vi "comicvine.to.local_issue.vi"(8 "error in (no error)":errorcluster, 11 "cv_issue":T5) -> (0 "error out":errorcluster, 3 "local_issue":T1)   [LabVIEW 2024]
uses:
  definitions/comicvine_issue.ctl
  definitions/comicvine_issue.results.ctl
  definitions/comicvine_issue.associated_image.ctl
  definitions/comicvine_issue.generic_credit.ctl
  definitions/comicvine_issue.person_credit.ctl
  definitions/local_issue.ctl
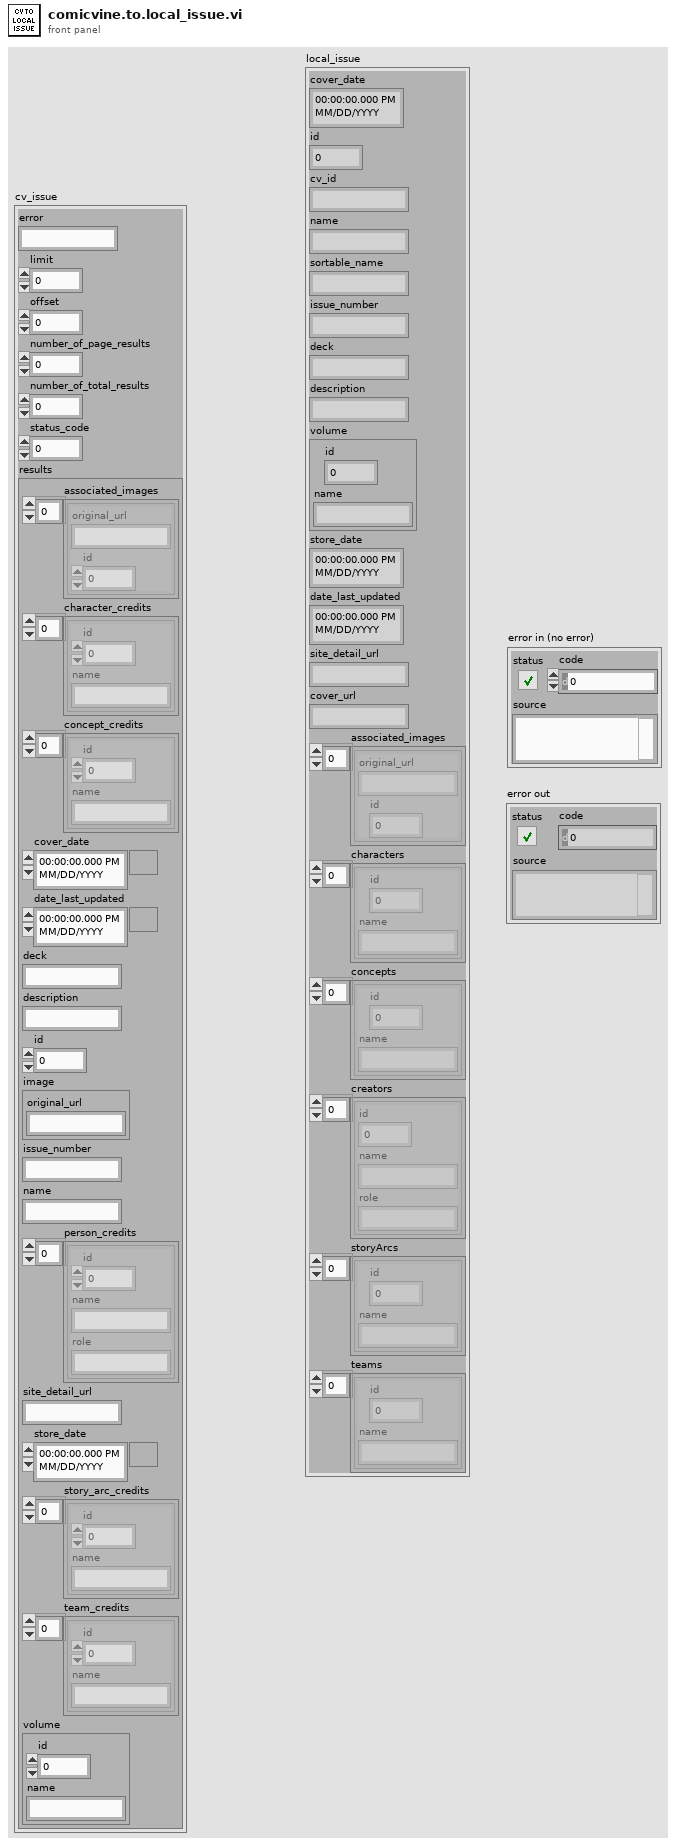
[diagram p1: front panel]
types:
  T1 = typedef "local_issue.ctl" = cluster{"cover_date":timestamp, "id":i32, "cv_id":string, "name":string, "sortable_name":string, "issue_number":string, "deck":string, "description":string, "volume":T2, "store_date":timestamp, "date_last_updated":timestamp, "site_detail_url":string, "cover_url":string, "associated_images":T3[], "characters":T2[], "concepts":T2[], "creators":T4[], "storyArcs":T2[], "teams":T2[]}
  T2 = typedef "comicvine_issue.generic_credit.ctl" = cluster{"id":i32, "name":string}
  T3 = typedef "comicvine_issue.associated_image.ctl" = cluster{"original_url":string, "id":i32}
  T4 = typedef "comicvine_issue.person_credit.ctl" = cluster{"id":i32, "name":string, "role":string}
  T5 = typedef "comicvine_issue.ctl" = cluster{"error":string, "limit":i32, "offset":i32, "number_of_page_results":i32, "number_of_total_results":i32, "status_code":i32, "results":T6}
  T6 = typedef "comicvine_issue.results.ctl" = cluster{"associated_images":T3[], "character_credits":T2[], "concept_credits":T2[], "cover_date":timestamp, "date_last_updated":timestamp, "deck":string, "description":string, "id":i32, "image":cluster{"original_url":string}, "issue_number":string, "name":string, "person_credits":T4[], "site_detail_url":string, "store_date":timestamp, "story_arc_credits":T2[], "team_credits":T2[], "volume":T2}
  T7 = typedef "LVDateTimeRec.ctl" = cluster{"fractional second":dbl, "second":i32, "minute":i32, "hour":i32, "day of month":i32, "month":i32, "year":i32, "day of week":i32, "day of year":i32, "DST":i32}
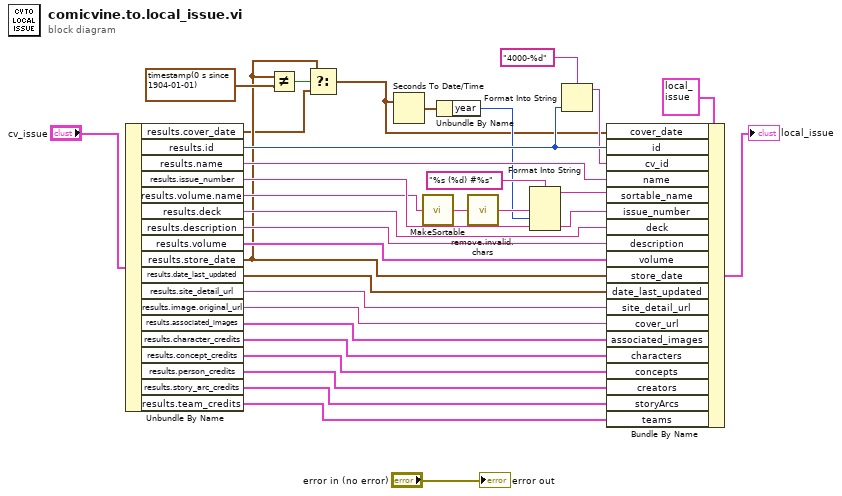
[diagram p0: block diagram]
diagram:
  n1 = Unbundle By Name("cv_issue") -> ("results.cover_date"=w2:timestamp, "results.id"=w29:i32, "results.name"=w24:string, "results.issue_number"=w20:string, "results.volume.name"=w6:string, "results.deck"=w19:string, "results.description"=w18:string, "results.volume"=w17:T2, "results.store_date"=w3:timestamp, "results.date_last_updated"=w16:timestamp, "results.site_detail_url"=w15:string, "results.image.original_url"=w14:string, "results.associated_images"=w13:T3[], "results.character_credits"=w12:T2[], "results.concept_credits"=w11:T2[], "results.person_credits"=w10:T4[], "results.story_arc_credits"=w9:T2[], "results.team_credits"=w8:T2[])
  n2 = Not Equal?(x=w3, y=timestamp(0 s since 1904-01-01)) -> (x != y?=w4:bool)
  n3 = Select(t=w3, s=w4, f=w2) -> (s? t:f=w1:timestamp)
  n4 = Seconds To Date/Time(time stamp (now)=w1) -> (date time rec=w22:T7)  [unwired: 1 in]
  n5 = call "MakeSortable.vi"("string in"=w6) -> ("string out"=w27:string)
  n6 = Unbundle By Name(w22) -> ("year"=w21:i32)
  n7 = call "remove.invalid.chars.vi"("string in"=w27) -> ("string out"=w25:string)
  n8 = Format Into String(format string="%s (%d) #%s", w25, w21, w20) -> (resulting string=w23:string)  [unwired: 2 in, 1 out]
  n9 = Format Into String(format string="4000-%d", w29) -> (resulting string=w28:string)  [unwired: 2 in, 1 out]
  n10 = Bundle By Name(cluster=T1 {"cover_date"=timestamp(0 s since 1904-01-01), "id"=0, "cv_id"="", "name"="", "sortable_name"="", "issue_number"="", "deck"="", "description"="", "volume"={"id"=0, "name"=""}, "store_date"=timestamp(0 s since 1904-01-01), "date_last_updated"=timestamp(0 s since 1904-01-01), "site_detail_url"="", "cover_url"="", "associated_images"=[], "characters"=[], "concepts"=[], "creators"=[], "storyArcs"=[], "teams"=[]} ("local_issue"), "cover_date"=w1, "id"=w29, "cv_id"=w28, "name"=w24, "sortable_name"=w23, "issue_number"=w20, "deck"=w19, "description"=w18, "volume"=w17, "store_date"=w3, "date_last_updated"=w16, "site_detail_url"=w15, "cover_url"=w14, "associated_images"=w13, "characters"=w12, "concepts"=w11, "creators"=w10, "storyArcs"=w9, "teams"=w8) -> (→"local_issue":T1)
  "error out" <- "error in (no error)"
